vi "PI_GCS3_Sample_Application_2_Controllers.vi"() -> ()   [LabVIEW 2026]
doc: "This VI demonstrates how to initialize two PI GCS3 systems and how to query the help answers. \nThe diagram shows how to combine the driver VIs for these tasks. \n\nWarning: Before running this VI, modify the interface settings on the block diagram to reflect your configuration. The predefined settings provided with the VI probably do not match your system."
uses:
  Low Level/Communication/Interface Settings.ctl
  Low Level/SpecialCommand/ModeOfOperation.ctl
panel:
  out "Help string Sys. 2":string
  out "Identification Sys. 2":string
  out "Connected Axis System 2":string[](array[string])
  out "Help string Sys. 1":string
  in  "stop":bool
  in  "error in":errorcluster
  out "Running":bool caption="Configuration_Setup.vis running"
  out "error out":errorcluster
  out "Connected Axis System 1":string[](array[string])
  out "Identification Sys. 1":string
  # "This VI demonstrates how to initialize two PI GCS3 systems and how to query their help answer. \nThe diagram shows how to combine the driver VIs for these tasks. \n\nWarning: Before running this VI, modify the interface settings on the block diagram to reflect your configuration. The predefined \n                 settings provided with the VI probably do not match your system."
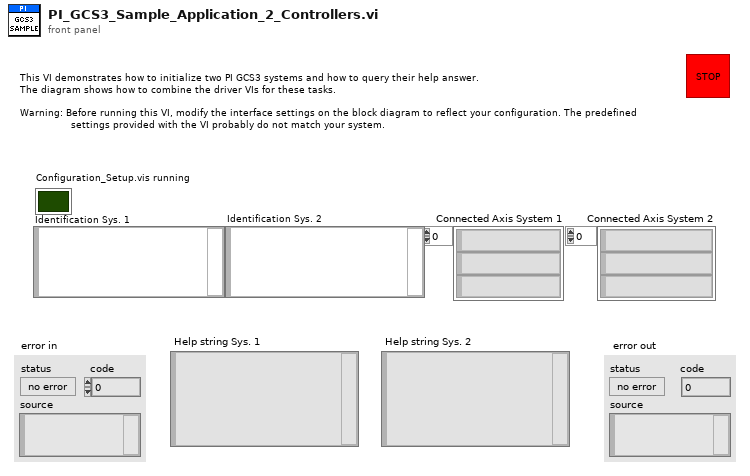
[diagram p1: front panel]
types:
  T1 = typedef "ModeOfOperation.ctl" = enum16{"Open", "Open-Loop Position", "Closed-Loop Position", "Open-Loop Velocity", "Closed-Loop Velocity", "Open-Loop Force", "Closed-Loop Force", "Step Operation"}
  T2 = typedef "Interface Settings.ctl" = cluster{"Interface":u16, "Timeout":u32, "RS232 settings":cluster{"Portnumber":u8, "Baudrate":u16}, "TCP/IP settings":cluster{"Host address/name":string, "Port":i32, "Board":i32, "TCP/IP Search?":bool}, "USB settings":cluster{"S/N":string, "USB Search?":bool}, "DaisyChain settings":cluster{"Register DC":bool, "DaisyChain Search?":bool, "Device ID":i32}, "DLL for Device":u16}
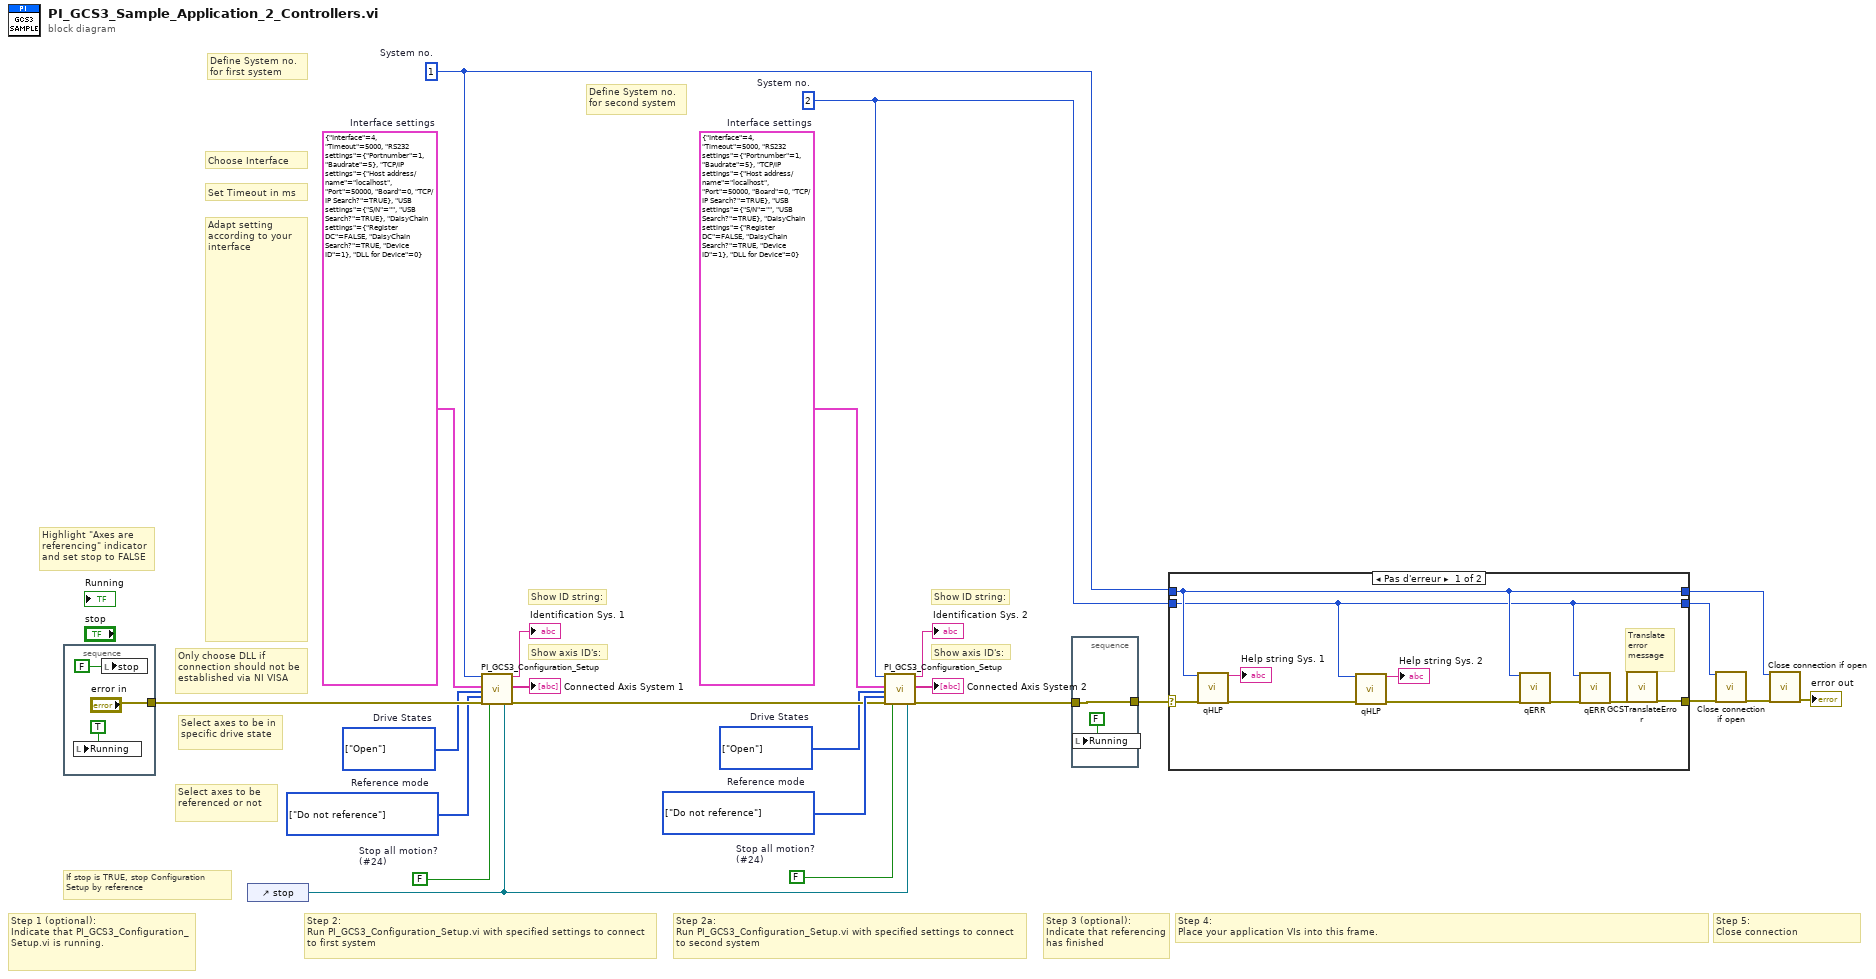
[diagram p0: block diagram]
diagram:
  w17 = enum16{"Do not reference", "Reference switch"}[] [enum."Do not reference"] items=["Do not reference", "Reference switch"]  # Reference mode
  w1 = T1[] [enum."Open"] items=["Open", "Open-Loop Position", "Closed-Loop Position", "Open-Loop Velocity", "Closed-Loop Velocity", "Open-Loop Force", "Closed-Loop Force", "Step Operation"]  # Drive States
  w5 = T1[] [enum."Open"] items=["Open", "Open-Loop Position", "Closed-Loop Position", "Open-Loop Velocity", "Closed-Loop Velocity", "Open-Loop Force", "Closed-Loop Force", "Step Operation"]  # Drive States
  w4 = enum16{"Do not reference", "Reference switch"}[] [enum."Do not reference"] items=["Do not reference", "Reference switch"]  # Reference mode
  w8 = T2 {"Interface"=4, "Timeout"=5000, "RS232 settings"={"Portnumber"=1, "Baudrate"=5}, "TCP/IP settings"={"Host address/name"="localhost", "Port"=50000, "Board"=0, "TCP/IP Search?"=TRUE}, "USB settings"={"S/N"="", "USB Search?"=TRUE}, "DaisyChain settings"={"Register DC"=FALSE, "DaisyChain Search?"=TRUE, "Device ID"=1}, "DLL for Device"=0}  # Interface settings
  w9 = T2 {"Interface"=4, "Timeout"=5000, "RS232 settings"={"Portnumber"=1, "Baudrate"=5}, "TCP/IP settings"={"Host address/name"="localhost", "Port"=50000, "Board"=0, "TCP/IP Search?"=TRUE}, "USB settings"={"S/N"="", "USB Search?"=TRUE}, "DaisyChain settings"={"Register DC"=FALSE, "DaisyChain Search?"=TRUE, "Device ID"=1}, "DLL for Device"=0}  # Interface settings
  w18 = FALSE  # Stop all motion? (#24)
  w7 = 2  # System no.
  w19 = FALSE  # Stop all motion? (#24)
  w6 = 1  # System no.
  # "Step 2a: \nRun PI_GCS3_Configuration_Setup.vi with specified settings to connect to second system"
  # "Define System no. for second system"
  # "Show axis ID's:"
  # "Show ID string:"
  # "Step 5: \nClose connection"
  # "Define System no.\nfor first system"
  # "Select axes to be referenced or not"
  # "Select axes to be in specific drive state"
  # "Adapt setting according to your interface"
  # "Set Timeout in ms"
  # "Choose Interface"
  # "Only choose DLL if connection should not be established via NI VISA"
  # "If stop is TRUE, stop Configuration\nSetup by reference"
  # "Step 4: \nPlace your application VIs into this frame."
  # "Step 3 (optional): \nIndicate that referencing has finished"
  # "Step 2: \nRun PI_GCS3_Configuration_Setup.vi with specified settings to connect to first system"
  # "Step 1 (optional): \nIndicate that PI_GCS3_Configuration_Setup.vi is running."
  # "Highlight \"Axes are\nreferencing\" indicator\nand set stop to FALSE"
  # "Show axis ID's:"
  # "Show ID string:"
  n1 = stacked-sequence {
    tunnel: ["error in"] -> w23
    frame #0 {
      n2 = local write "Running"(TRUE ("Running")) -> ()
      n3 = local write "stop"(FALSE ("stop")) -> ()
    }
  }
  n4 = control-ref of="stop"() -> (w13:refnum<vi>)
  n5 = call "PI_GCS3_Configuration_Setup.vi"("System no."=w6, "Interface settings"=w9, "Mode of operation"=w5, "Reference mode"=w4, "error in"=w23, "Stop all motion?"=w19, "Stop refnum"=w13) -> ("Identification"=→"Identification Sys. 1":string, "Conn. axis"=→"Connected Axis System 1":string[], "error out"=w14:errorcluster)  [unwired: 7 in, 3 out]
  n6 = call "PI_GCS3_Configuration_Setup.vi"("System no."=w7, "Interface settings"=w8, "Mode of operation"=w1, "Reference mode"=w17, "error in"=w14, "Stop all motion?"=w18, "Stop refnum"=w13) -> ("Identification"=→"Identification Sys. 2":string, "Conn. axis"=→"Connected Axis System 2":string[], "error out"=w12:errorcluster)  [unwired: 7 in, 3 out]
  n7 = stacked-sequence {
    tunnel: w12 -> [w28]
    tunnel: [w28] -> w22
    frame #0 {
      n8 = local write "Running"(FALSE ("Running")) -> ()
    }
  }
  n9 = case shown="Pas d'erreur" w22 {
    selector: w22 -> [w37 w41]
    tunnel: [w38 w41] -> w11
    tunnel: w6 -> [w31 w40]
    tunnel: w7 -> [w30 w39]
    tunnel: [w31 w40] -> w2
    tunnel: [w30 w39] -> w3
    frame No Error {
      # "Translate\nerror \nmessage"
      n10 = call "qHLP.vi"("System no."=w31, "error in"=w37) -> ("Help string"=→"Help string Sys. 1":string, "error out"=w36:errorcluster)  [unwired: 16 out]
      n11 = call "qHLP.vi"("System no."=w30) -> ("Help string"=→"Help string Sys. 2":string)  [unwired: 1 in, 17 out]
      n12 = call "qERR.vi"("System no."=w31, "error in"=w36) -> ("error out"=w33:errorcluster)  [unwired: 17 out]
      n13 = call "qERR.vi"("System no."=w30, "error in"=w33) -> ("error out"=w32:errorcluster)  [unwired: 17 out]
      n14 = call "GCSTranslateError.vi"("error in"=w32) -> ("error out"=w38:errorcluster)  [unwired: 18 out]
    }
    frame Error {
      # "Error during initialization"
    }
  }
  n15 = call "Close connection if open.vi"("System no."=w3, "error in"=w11) -> ("error out"=w10:errorcluster)  [unwired: 1 in, 16 out]
  n16 = call "Close connection if open.vi"("System no."=w2, "error in"=w10) -> ("error out"=→"error out":errorcluster)  [unwired: 1 in, 16 out]
